vi "FTW-CodeGen-RelinkTerminals.vi"(0 "Diagram":refnum<vi>, 5 "Terms":T1(array[cluster]), 7 "PrototypeVI":refnum<vi>, 11 "error in":errorcluster) -> (4 "Diagram out":refnum<vi>, 15 "error out":errorcluster)   [LabVIEW 2015]
uses:
  src/error/FTW-ERR-NoErrorConstant.vi
  lib/FTW-KernelFilepath.vi
panel:
  out "Relink":dbl format="%.6psec"
  out "Move":dbl format="%.6psec"
  # "Inputs"
  # "Outputs"
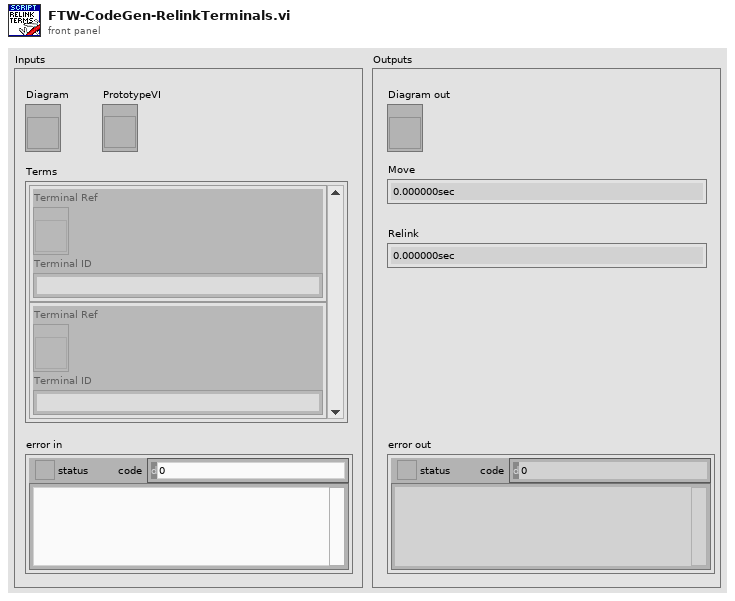
[diagram p1: front panel]
types:
  T1 = cluster{"Terminal Ref":refnum<vi>, "Terminal ID":string}[]
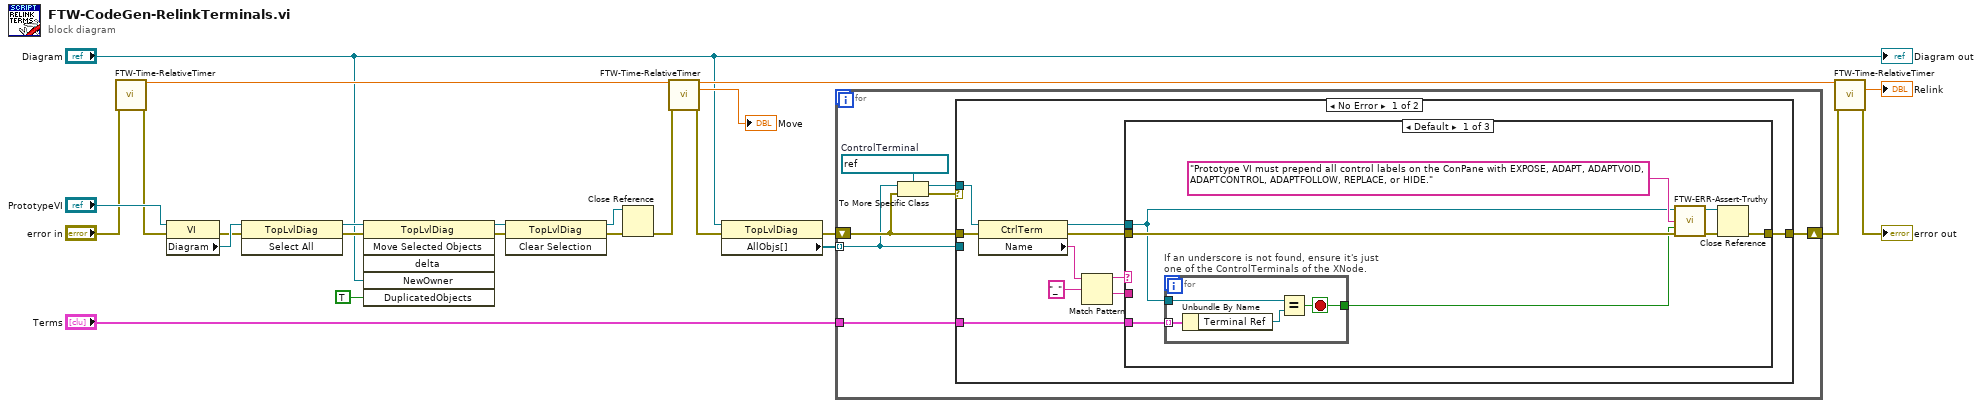
[diagram p0: block diagram]
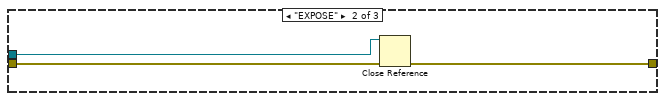
[diagram p2: hidden frame]
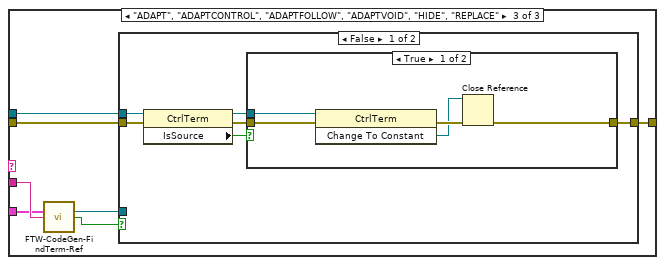
[diagram p3: hidden frame]
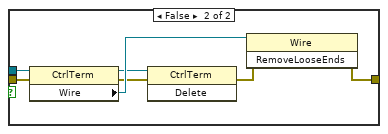
[diagram p4: hidden frame]
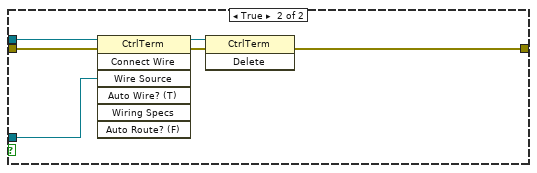
[diagram p5: hidden frame]
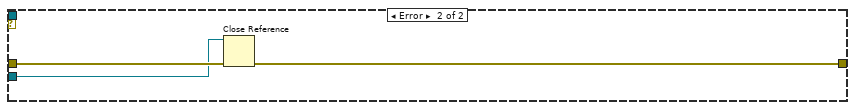
[diagram p6: hidden frame]
diagram:
  n1 = call "FTW-Time-RelativeTimer.vi"("error in"="error in") -> ("Current Timer Value"=w10:dbl, "error out"=w17:errorcluster)  [unwired: 12 in, 1 out]
  n2 = property class="VI"(reference="PrototypeVI", error in=w17) -> (error out=w21:errorcluster, "Diagram"=w22:refnum<vi>)  [unwired: 1 out]
  n3 = invoke class="TopLvlDiag" method="Select All"(reference=w22, error in=w21) -> (reference out=w23:refnum<vi>, error out=w9:errorcluster)  [unwired: 1 in, 1 out]
  n4 = invoke class="TopLvlDiag" method="Move Selected Objects"(reference=w23, error in=w9, "NewOwner"="Diagram", "DuplicatedObjects"=TRUE ("Duplicate? (F)")) -> (reference out=w7:refnum<vi>, error out=w1:errorcluster)  [unwired: 2 in, 4 out]
  n5 = invoke class="TopLvlDiag" method="Clear Selection"(reference=w7, error in=w1) -> (reference out=w6:refnum<vi>, error out=w8:errorcluster)  [unwired: 1 in, 1 out]
  n6 = Close Reference(reference=w6, error in (no error)=w8) -> (error out=w16:errorcluster)
  n7 = call "FTW-Time-RelativeTimer.vi"("Previous Timer Value"=w10, "error in"=w16) -> ("Current Timer Value"=w14:dbl, "Elapsed Time"=→"Move":dbl, "error out"=w5:errorcluster)  [unwired: 11 in]
  n8 = property class="TopLvlDiag"(reference="Diagram", error in=w5) -> (error out=w4:errorcluster, "AllObjs[]"=w3:refnum<vi>[])  [unwired: 1 out]
  n9 = for {
    tunnel: w3 -> [w25] mode=indexing
    tunnel: "Terms" -> [w28]
    shift-right: [w30] -> w11
    shift-left: w4 -> [w26]
    w29 = refnum<vi> refnum  # ControlTerminal
    n10 = To More Specific Class(target class=w29, reference=w25, error in=w26) -> (specific class reference=w31:refnum<vi>, error out=w27:errorcluster)
    n11 = case shown="No Error" w27 {
      tunnel: w31 -> [w41 _]
      tunnel: [w40 w88] -> w30
      tunnel: w28 -> [w35 _]
      tunnel: w26 -> [w32 w89]
      tunnel: w25 -> [_ w87]
      frame No Error {
        n12 = property class="CtrlTerm"(reference=w41, error in=w32) -> (reference out=w39:refnum<vi>, error out=w38:errorcluster, "Name"=w33:string)
        n13 = Match Pattern(string=w33, regular expression="_") -> (before substring=w36:string, after substring=w34:string)  [unwired: 1 in, 2 out]
        n14 = case shown="Default" w36 {
          tunnel: w39 -> [w44 w54 w62]
          tunnel: w38 -> [w45 w55 w61]
          tunnel: [w46 w53 w60] -> w40
          tunnel: w35 -> [w43 _ w56]
          tunnel: w34 -> [_ _ w57]
          frame Default {
            n15 = for "If an underscore is not found, ensure it's just one of the ControlTerminals of the XNode." {
              tunnel: [w52] -> w42
              tunnel: w43 -> [w51] mode=indexing
              tunnel: w44 -> [w49]
              stop <- w52 stop-if-true
              n16 = Unbundle By Name(w51) -> ("Terminal Ref"=w50:refnum<vi>)
              n17 = Equal?(x=w49, y=w50) -> (x = y?=w52:bool)
            }
            n18 = call "FTW-ERR-Assert-Truthy.vi"("Assertion"="Prototype VI must prepend all control labels on the ConPane with EXPOSE, ADAPT, ADAPTVOID, ADAPTCONTROL, ADAPTFOLLOW, REPLACE, or HIDE.", "Assertion holds true?"=w42, "error in"=w45) -> ("error out"=w47:errorcluster)  [unwired: 12 in]
            n19 = Close Reference(reference=w44, error in (no error)=w47) -> (error out=w46:errorcluster)
          }
          frame "EXPOSE" {
            n20 = Close Reference(reference=w54, error in (no error)=w55) -> (error out=w53:errorcluster)
          }
          frame "ADAPT", "ADAPTCONTROL", "ADAPTFOLLOW", "ADAPTVOID", "HIDE", "REPLACE" {
            n21 = call "FTW-CodeGen-FindTerm-Ref.vi"("Terms"=w56, "Terminal ID"=w57) -> ("Terminal Ref"=w59:refnum<vi>, "Found?"=w58:bool)  [unwired: 12 in]
            n22 = case shown="False" w58 {
              tunnel: w59 -> [_ w83]
              tunnel: w62 -> [w63 w86]
              tunnel: w61 -> [w67 w85]
              tunnel: [w68 w84] -> w60
              frame False {
                n23 = property class="CtrlTerm"(reference=w63, error in=w67) -> (reference out=w66:refnum<vi>, error out=w64:errorcluster, "IsSource"=w65:bool)
                n24 = case shown="True" w65 {
                  tunnel: [w69 w78] -> w68
                  tunnel: w66 -> [w72 w80]
                  tunnel: w64 -> [w73 w79]
                  frame True {
                    n25 = invoke class="CtrlTerm" method="Change To Constant"(reference=w72, error in=w73) -> (error out=w71:errorcluster, "Change To Constant"=w70:refnum<vi>)  [unwired: 1 in, 1 out]
                    n26 = Close Reference(reference=w70, error in (no error)=w71) -> (error out=w69:errorcluster)
                  }
                  frame False {
                    n27 = property class="CtrlTerm"(reference=w80, error in=w79) -> (reference out=w76:refnum<vi>, error out=w75:errorcluster, "Wire"=w77:refnum<vi>)
                    n28 = invoke class="CtrlTerm" method="Delete"(reference=w76, error in=w75) -> (error out=w74:errorcluster)  [unwired: 1 in, 2 out]
                    n29 = invoke class="Wire" method="RemoveLooseEnds"(reference=w77, error in=w74) -> (error out=w78:errorcluster)  [unwired: 1 in, 2 out]
                  }
                }
              }
              frame True {
                n30 = invoke class="CtrlTerm" method="Connect Wire"(reference=w86, error in=w85, "Wire Source"=w83) -> (reference out=w82:refnum<vi>, error out=w81:errorcluster)  [unwired: 4 in, 5 out]
                n31 = invoke class="CtrlTerm" method="Delete"(reference=w82, error in=w81) -> (error out=w84:errorcluster)  [unwired: 1 in, 2 out]
              }
            }
          }
        }
      }
      frame Error {
        n32 = Close Reference(reference=w87, error in (no error)=w89) -> (error out=w88:errorcluster)
      }
    }
  }
  n33 = call "FTW-Time-RelativeTimer.vi"("Previous Timer Value"=w14, "error in"=w11) -> ("Elapsed Time"=→"Relink":dbl, "error out"=→"error out":errorcluster)  [unwired: 11 in, 1 out]
  "Diagram out" <- "Diagram"
